vi "TSM Get Low Noise Mic Settings.vi"(0 "TSM context":T1, 11 "error in (no error)":errorcluster) -> (4 "TSM context Out":T1, 6 "Sampling Rate (Hz)":dbl format="%#_13g", 8 "Samples per channel":i32=1000, 15 "error out":errorcluster)   [LabVIEW 2020]
doc: "Get the settings from Spec sheet using TSM context"
uses:
  <vilib>/NI_TestStand_SemiconductorModule/NI_TestStand_Semiconductor_Module.lvlibp/PinMap/General/SemiconductorModuleContext.ctl
  <vilib>/NI_TestStand_SemiconductorModule/NI_TestStand_Semiconductor_Module.lvlibp/PinMap/Specs/NamespacedSymbolsToValues.vi
  <vilib>/NI_TestStand_SemiconductorModule/NI_TestStand_Semiconductor_Module.lvlibp
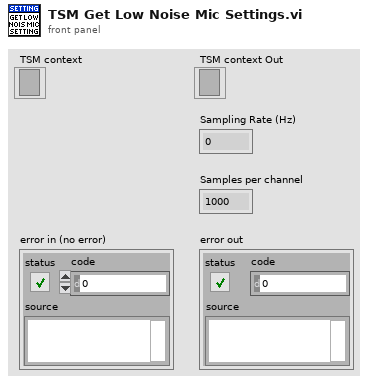
[diagram p1: front panel]
types:
  T1 = typedef "NI_TestStand_Semiconductor_Module.lvlibp/SemiconductorModuleContext.ctl" = refnum<k7>
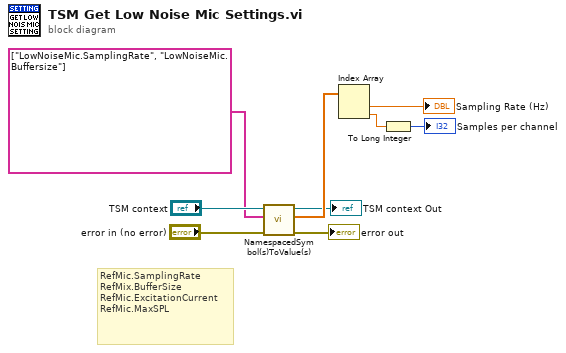
[diagram p0: block diagram]
diagram:
  # "RefMic.SamplingRate\nRefMix.BufferSize\nRefMic.ExcitationCurrent\nRefMic.MaxSPL"
  n1 = call-poly <vilib>:"NamespacedSymbol(s)ToValue(s).vi"("error in (no error)"="error in (no error)", "Symbols"=tag[] ["LowNoiseMic.SamplingRate", "LowNoiseMic.Buffersize"], "Semiconductor Module Context"="TSM context") -> ("error out"=→"error out":errorcluster, "Values"=w6:dbl[], "Semiconductor Module Context Out"=→"TSM context Out":T1)  [unwired: 6 in]
  n2 = Index Array(array=w6) -> (element #1=→"Sampling Rate (Hz)":dbl, element #2=w1:dbl)  [unwired: 2 in]
  n3 = To Long Integer(number=w1) -> (32bit integer=→"Samples per channel":i32)
